vi "Open Door.vi"(8 "error in (no error)":errorcluster, 11 "Doors Open in":refnum<class "Doors Open.lvclass">) -> (0 "error out":errorcluster, 3 "Doors Open out":refnum<class "Doors Open.lvclass">)   [LabVIEW 2020, in "Door Controller.lvlib" / "Doors Open.lvclass"]
uses:
  Doors Open.lvclass
  Doors Open.lvclass/Doors Open.ctl
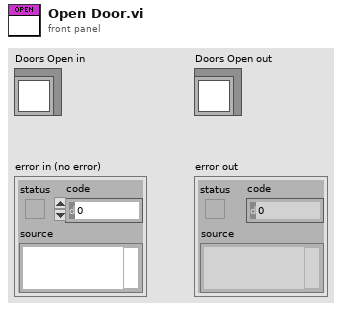
[diagram p1: front panel]
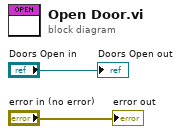
[diagram p0: block diagram]
diagram:
  "error out" <- "error in (no error)"
  "Doors Open out" <- "Doors Open in"
